vi "Square Root Calculator.vi"() -> ()   [LabVIEW 2017]
panel:
  out "root x":dbl
  in  "x":dbl
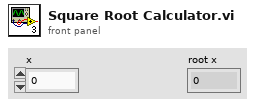
[diagram p1: front panel]
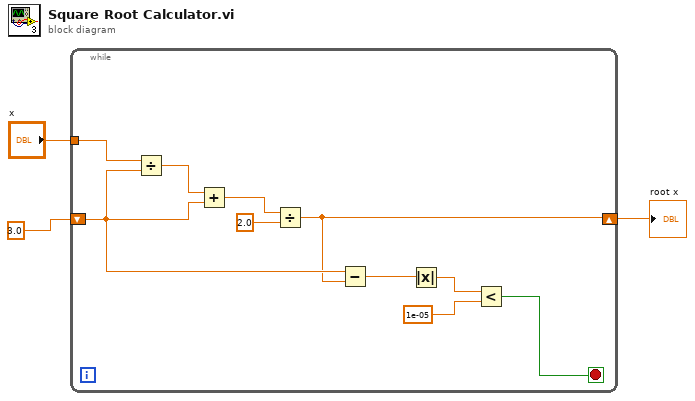
[diagram p0: block diagram]
diagram:
  n1 = while {
    shift-right: [w4] -> w1
    shift-left: 3.0 ("root x") -> [w9]
    tunnel: "x" -> [w13]
    stop <- w5 stop-if-true
    n2 = Divide(x=w13, y=w9) -> (x/y=w12:dbl)
    n3 = Add(x=w12, y=w9) -> (x+y=w11:dbl)
    n4 = Divide(x=w11, y=2.0) -> (x/y=w4:dbl)
    n5 = Subtract(x=w9, y=w4) -> (x-y=w8:dbl)
    n6 = Absolute Value(x=w8) -> (abs(x)=w7:dbl)
    n7 = Less?(x=w7, y=1e-05) -> (x < y?=w5:bool)
  }
  "root x" <- w1
